vi "GROUND cube sat.vi"() -> ()   [LabVIEW 2020]
uses:
  <vilib>/Utility/file.llb/Write Delimited Spreadsheet (string).vi
  <vilib>/Instr/_visa.llb/VISA Configure Serial Port (Instr).vi
panel:
  out "after BMP":string
  in  "read buffer":string
  in  "Tab Control":enum32{"Page 1", "Page 2"}(tab)
  out "Sensor ID":string
  out "SSTL":string
  out "AER":string
  in  "?":bool
  out "result":bool
  in  "?":T1(tab)
  out "RIGHT DATA":bool
  out "WRONG DATA":bool
  out "True password":bool
  in  "file path (dialog if empty) 2":path
  in  "VISA resource name":refnum<visa-resource-name>
  in  "Password":string
  in  "Username":string
  in  "OK":bool
  out "msg":string
  out "String":string
  in  "Send command":bool
  in  "velocity":dbl
  in  "distance":dbl
  out "time":dbl
  out "BMP Temprature (C)":dbl(slide) scale=0.0..100.0
  out "Altitude (m)":dbl(slide) scale=0.0..100000.0
  out "Pressure (Pa)":dbl(knob) scale=0.0..101325.0
  out "Altitude(m)":dbl
  out "Pressure(Pa)":dbl
  out "Temperature(C)":dbl
  out "Reads_BMP":string
  out "BMP_CRC WORKING":bool
  out "DHT temp (C)":dbl(slide) scale=-100.0..100.0
  out "DHT humidity (%)":dbl(knob) scale=0.0..100.0
  out "DHT temp(C)":dbl
  out "DHT humidity(%)":dbl
  out "Reads_DHT":string
  out "DHT_CRC WORKING":bool
  out "accel_z":dbl(slide) scale=0.0..1000.0
  out "accel_y":dbl(slide) scale=0.0..1000.0
  out "accel_x":dbl(slide) scale=0.0..1000.0
  out "phi":dbl(slide) scale=0.0..360.0
  out "theta":dbl(slide) scale=0.0..360.0
  out "psi":dbl(slide) scale=0.0..360.0
  out "FILTERD SIGNALS":dynamicdata(graph)
  out "SIGNALS":dynamicdata(graph)
  out "accel_x (m/s^2)":dbl
  out "accel_z(m/s^2)":dbl
  out "accel_y(m/s^2)":dbl
  out "phi":dbl
  out "psi":dbl
  out "theta":dbl
  in  "?":bool
  in  "Start Filtering":bool
  out "Reads_MPU":string
  out "MPU_CRC WORKING":bool
  out "ALT":i32
  in  "Zoom":sgl=16.0 format="%#.1g"
  in  "Size Y":dbl=650.0
  in  "Size X":dbl=450.0
  in  "Map Format":string(combo)="roadmap"
  out "LAT":i32
  out "LONG":i32
  in  "WebBrowser":refnum<k7>(container)
  out "ID":string
  out "Reads_GPS":string
  out "GPS_CRC WORKING":bool
  out "Image Out":T2(plugin-control)
  in  "Contrast::Value":dbl=0.32 min=0.0 max=0.64
  in  "Bayer::Gain R":dbl=1.0 min=0.0 max=3.999
  in  "Hue::Value":dbl min=-0.4 max=0.4
  in  "Bayer::Gain B":dbl=1.0 min=0.0 max=3.999
  in  "Bayer::Gain G":dbl=1.0 min=0.0 max=3.999
  out "pic number":dbl
  in  "Stop (F)":bool
  out "Time":string
  in  "Gamma::Value":dbl=1.0 min=0.72 max=5.0
  in  "Brightness::Value":i64 min=-64 max=64 step=1
  in  "Sharpness::Value":i64 min=0 max=5 step=1
  in  "Saturation::Value":i64=64 min=0 max=128 step=1
  in  "Take pic":bool
  in  "path":string
  # "The Cube sat"
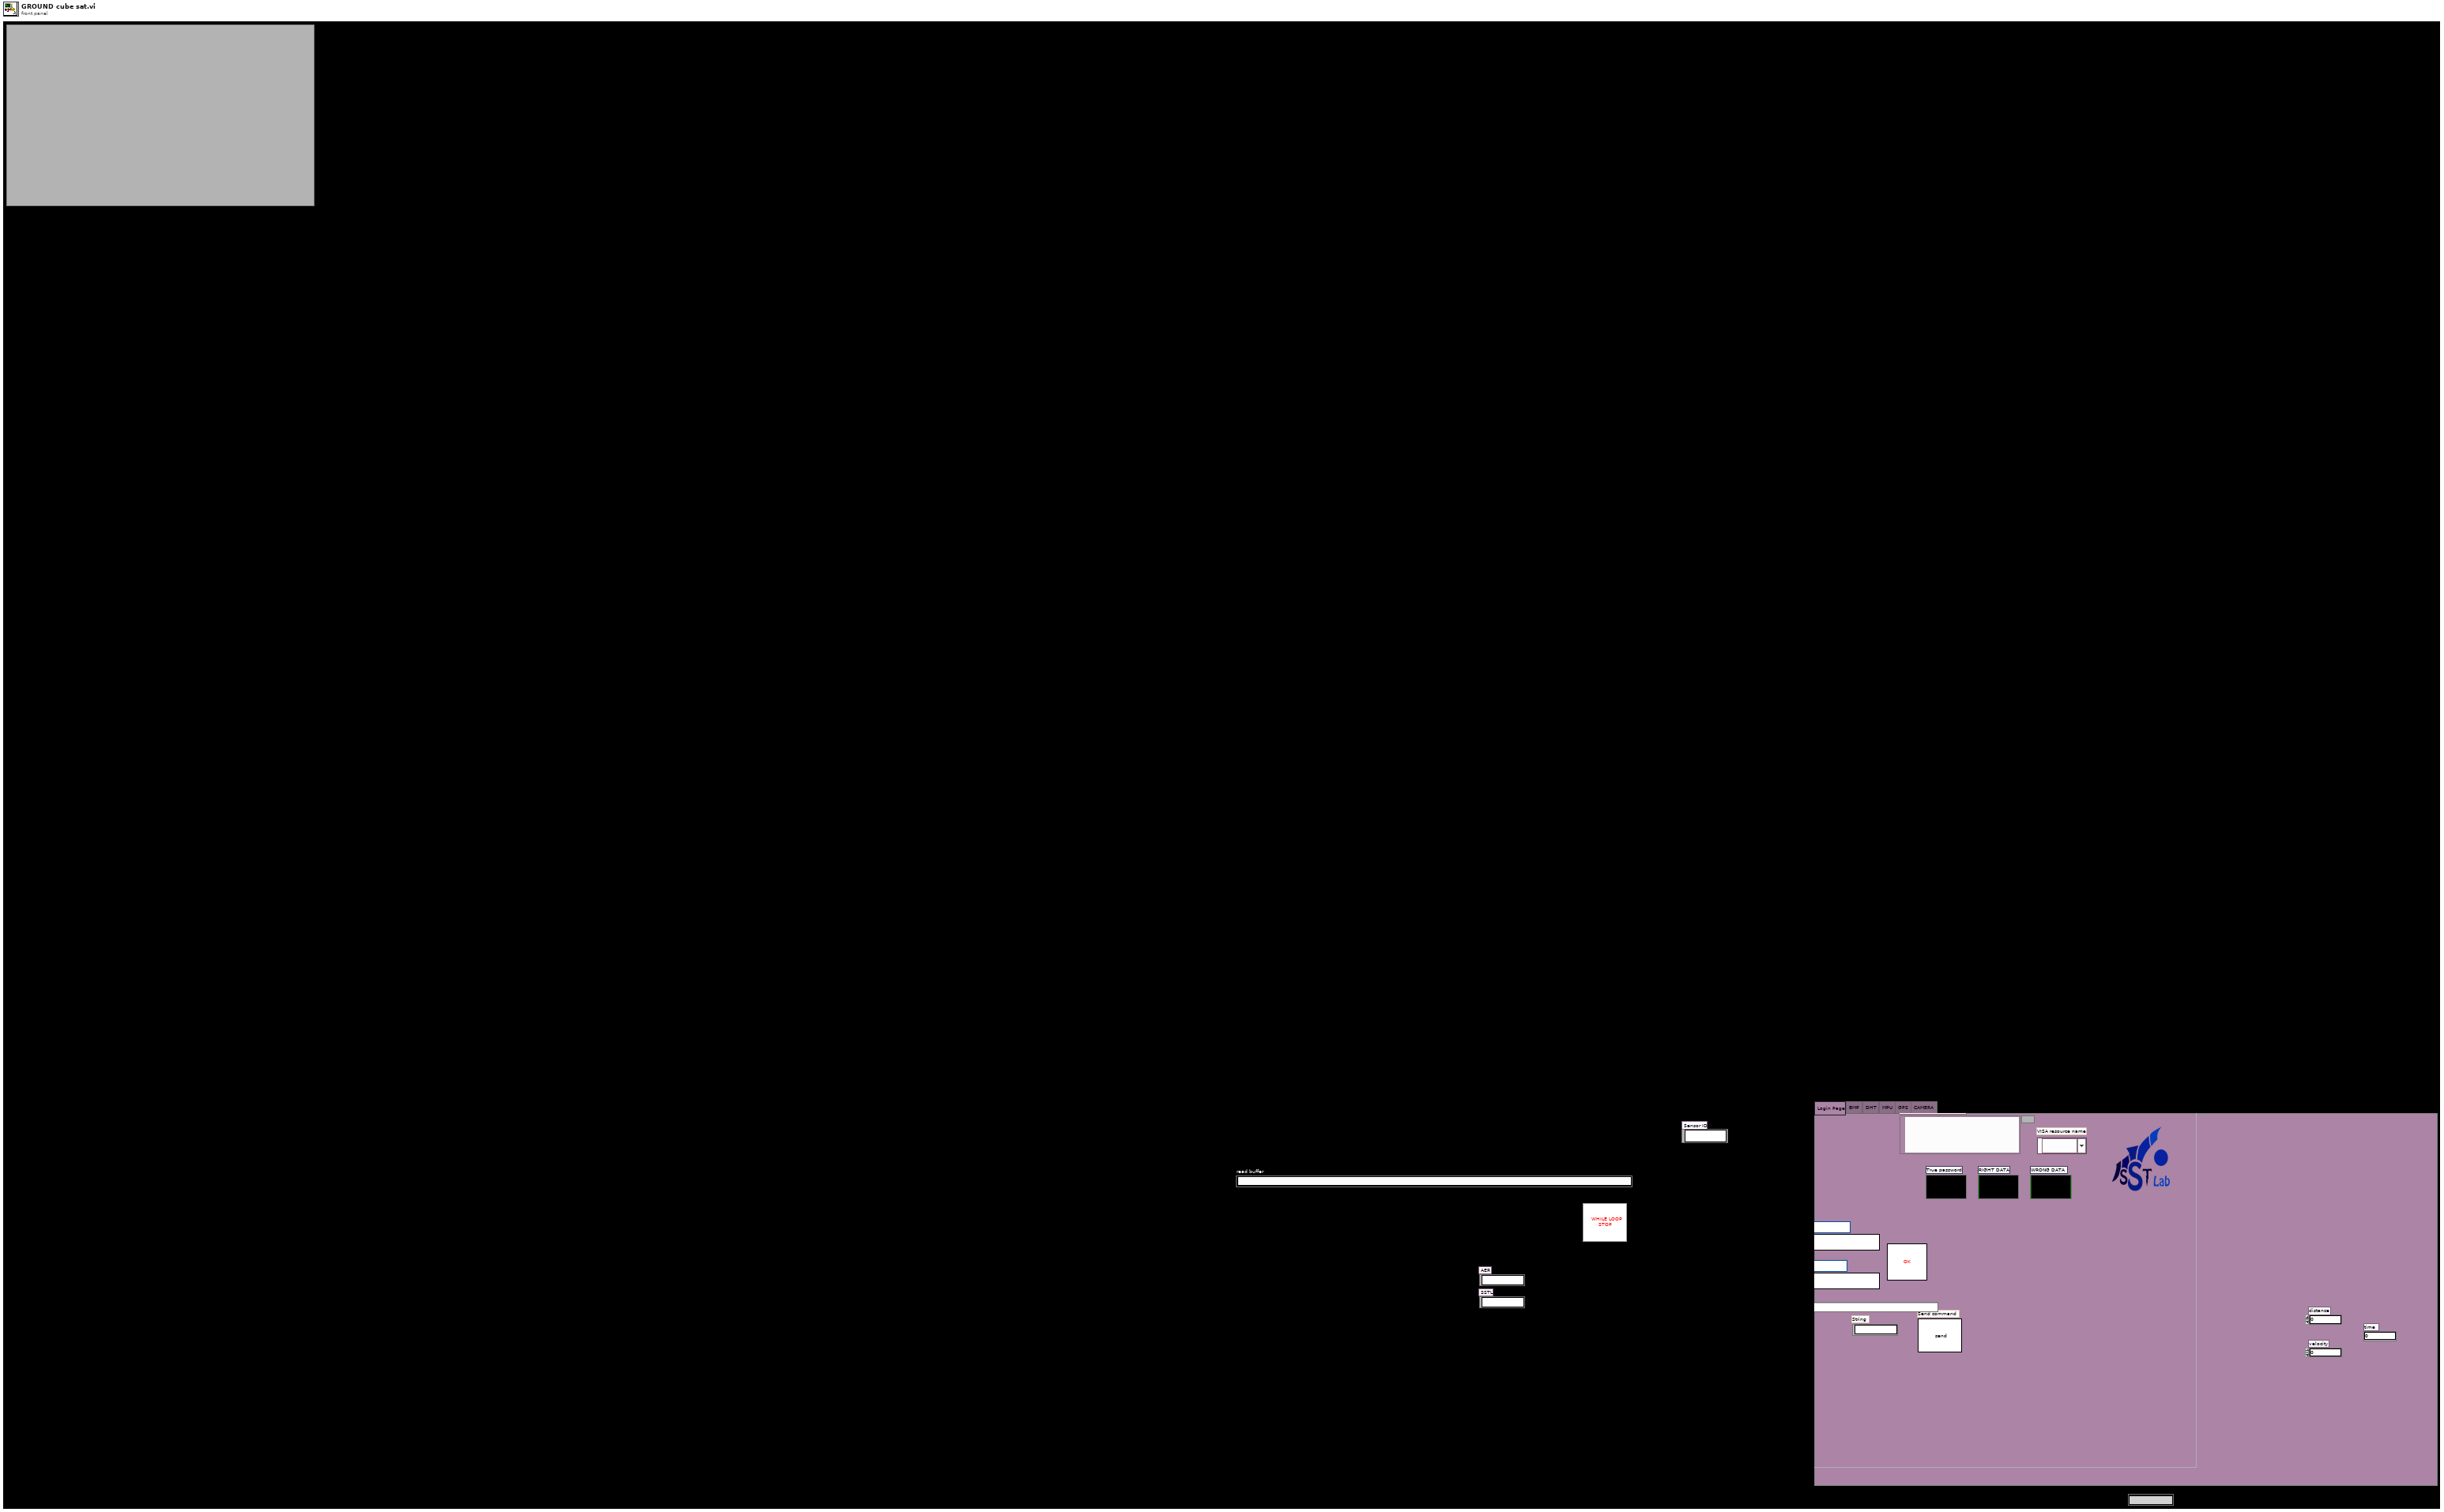
[diagram p1: front panel]
types:
  T1 = enum32{"Login Page", "BMP", "DHT", "MPU", "GPS", "CAMERA"}
  T2 = typedef "IMAQ Image.ctl" = refnum<image>
  T3 = enum32{"Page 1", "Page 2", "Page 3", "Page 4", "Page 5", "Page 6"}
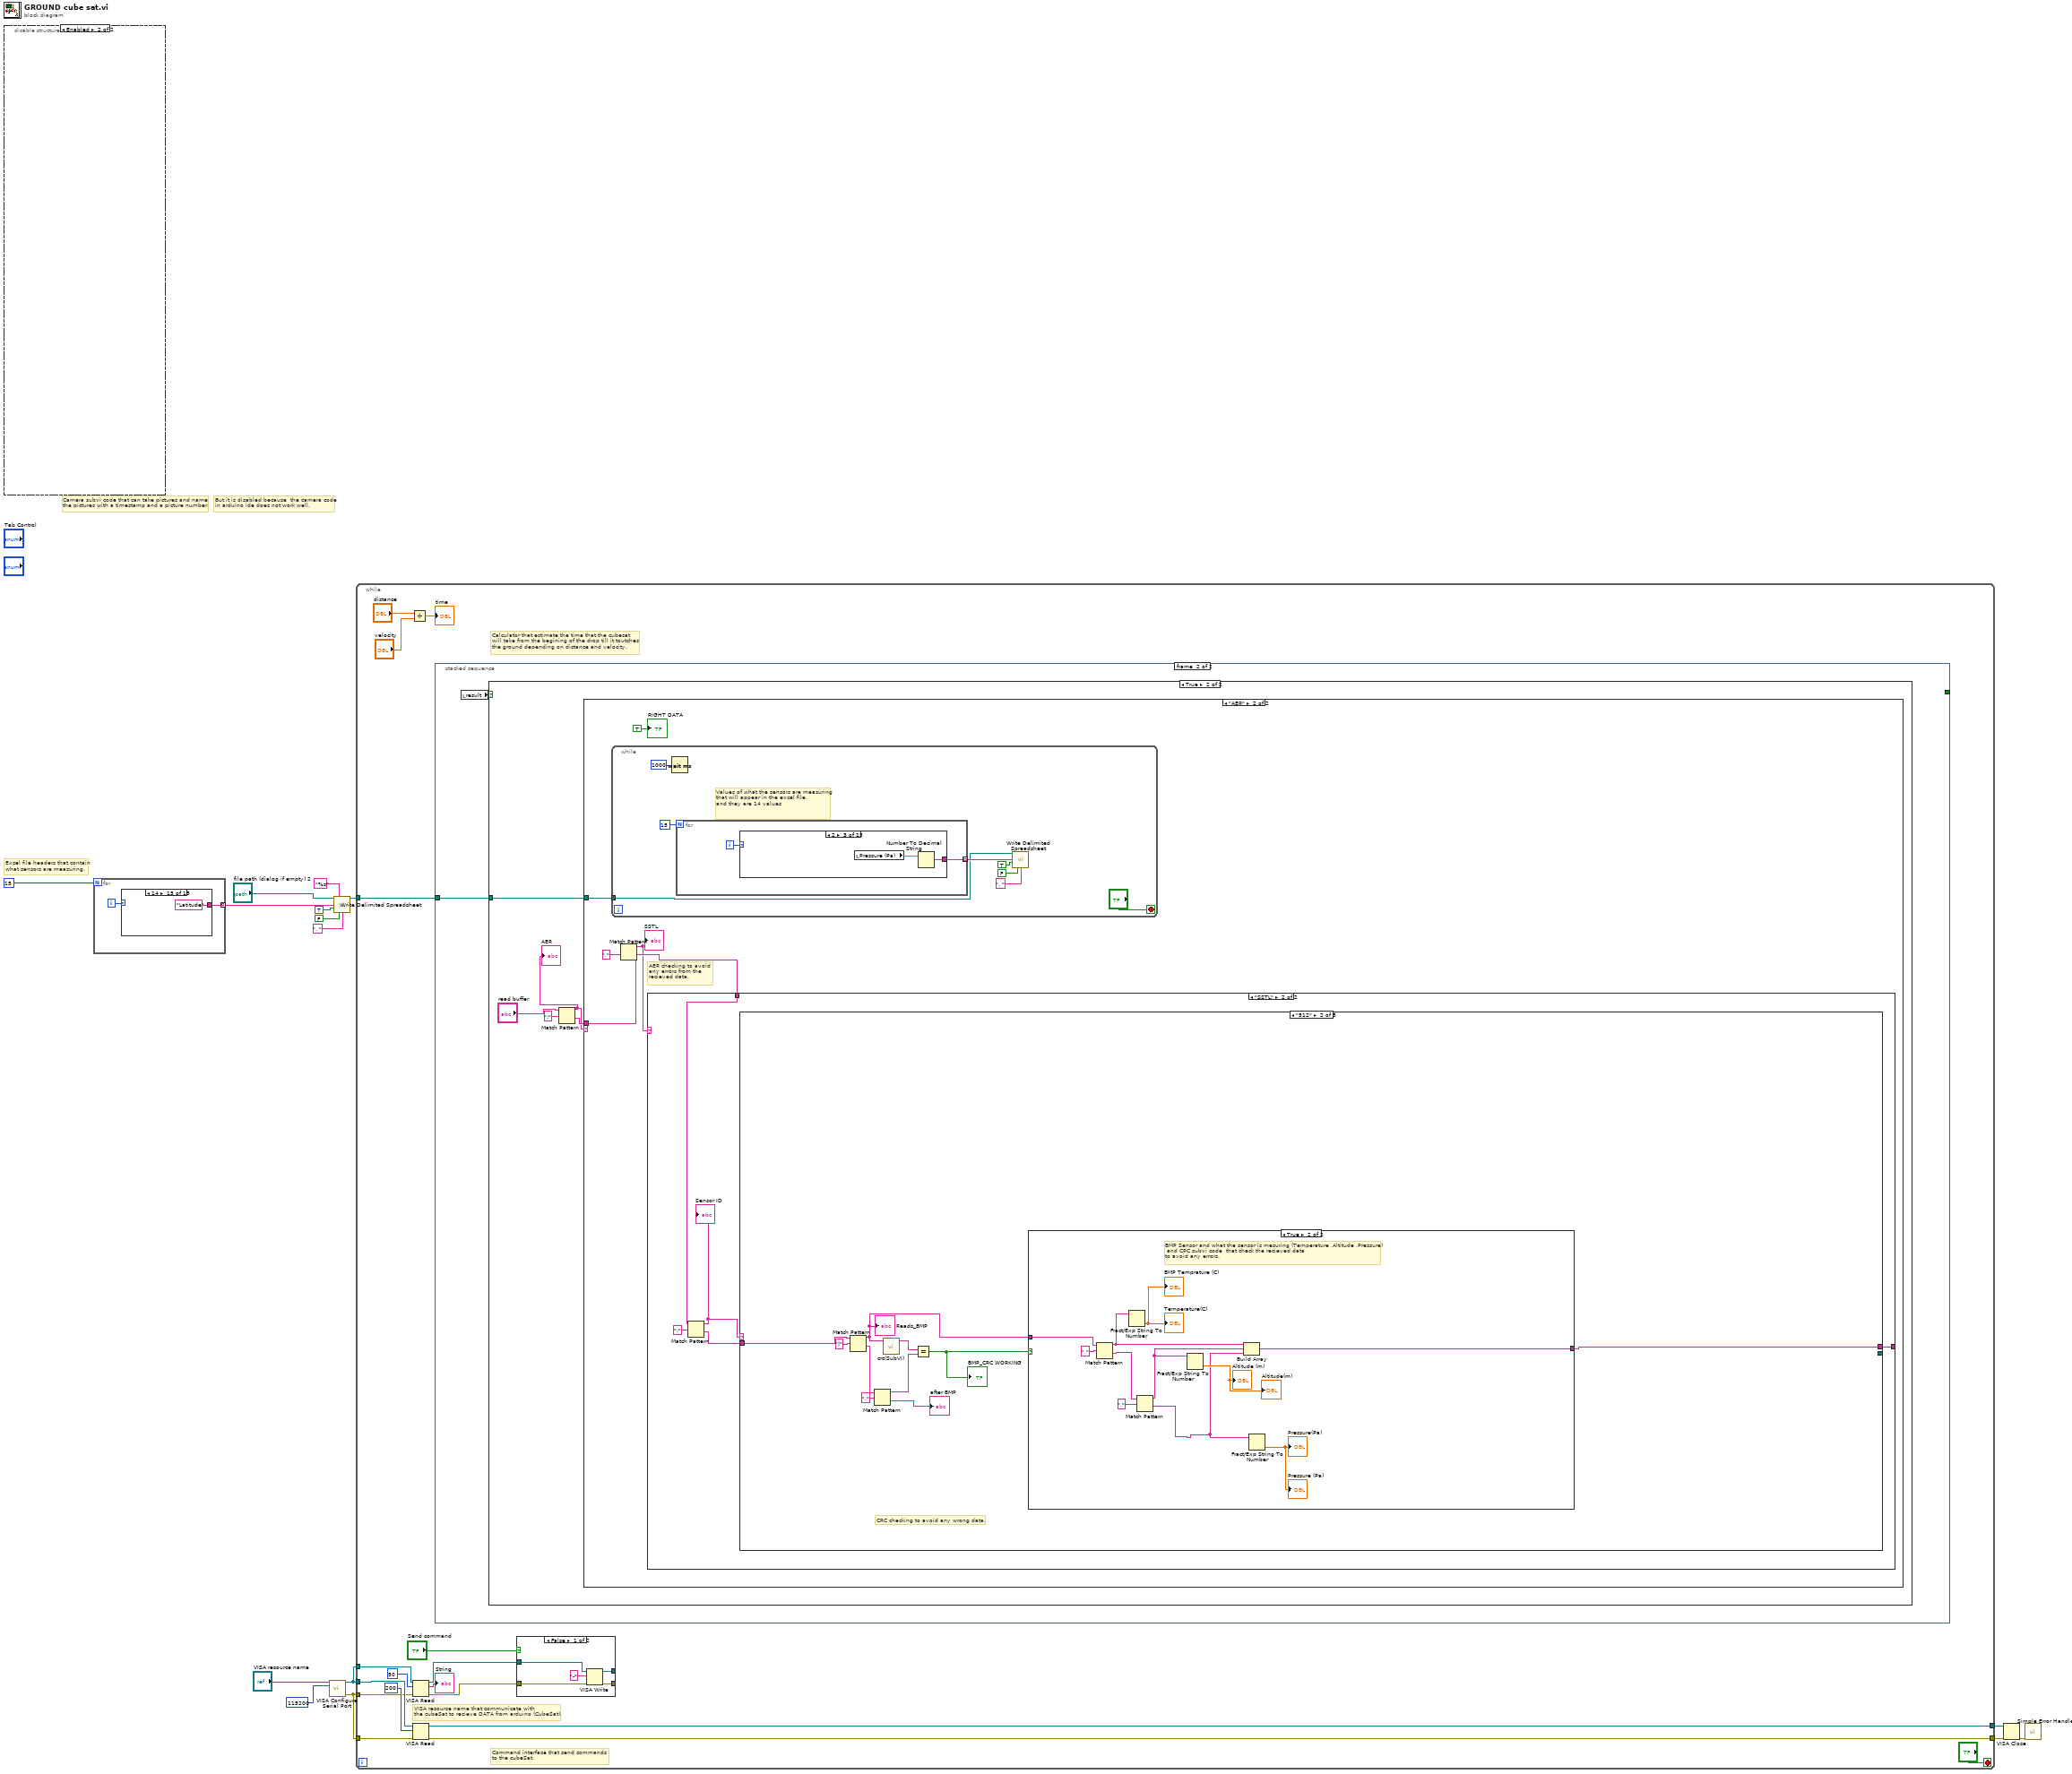
[diagram p0: block diagram]
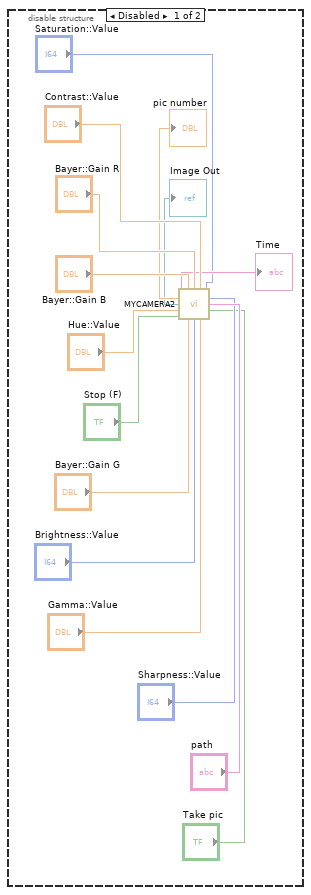
[diagram p2: hidden frame]
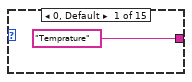
[diagram p3: hidden frame]
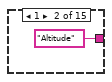
[diagram p4: hidden frame]
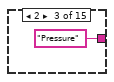
[diagram p5: hidden frame]
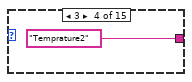
[diagram p6: hidden frame]
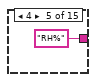
[diagram p7: hidden frame]
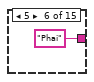
[diagram p8: hidden frame]
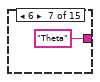
[diagram p9: hidden frame]
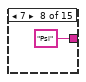
[diagram p10: hidden frame]
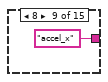
[diagram p11: hidden frame]
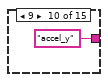
[diagram p12: hidden frame]
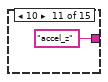
[diagram p13: hidden frame]
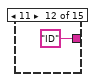
[diagram p14: hidden frame]
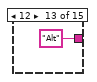
[diagram p15: hidden frame]
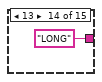
[diagram p16: hidden frame]
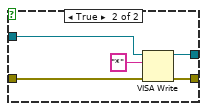
[diagram p17: hidden frame]
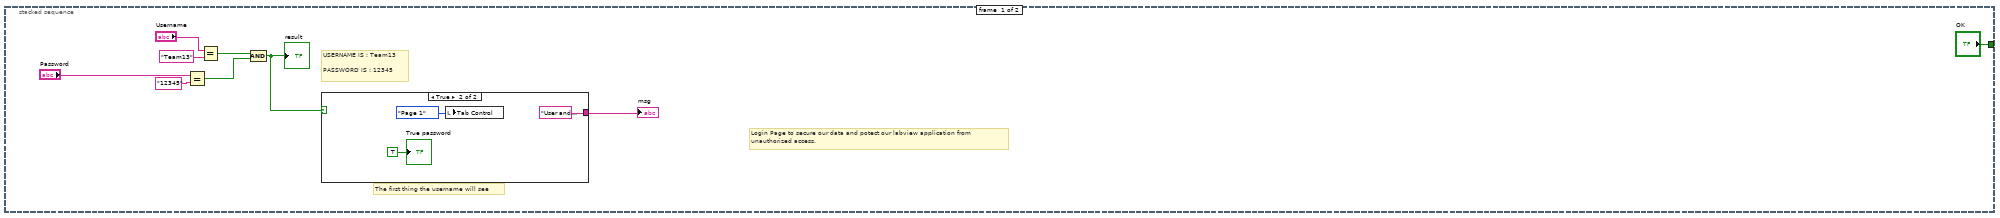
[diagram p18: hidden frame]
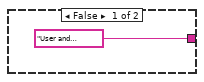
[diagram p19: hidden frame]
diagram:
  # "But it is disabled because  the camera code \nin arduino ide does not work well."
  # "Excel file headers that contain\nwhat sensors are measuring."
  # "Camera subvi code that can take pictures and name \nthe pictures with a timestamp and a picture number."
  n1 = disable-structure shown="Enabled" {
    frame Disabled {
      n2 = call "MYCAMERA2.vi"("Bayer::Gain B"="Bayer::Gain B", "Bayer::Gain R"="Bayer::Gain R", "Contrast::Value"="Contrast::Value", "Saturation::Value"="Saturation::Value", "Sharpness::Value"="Sharpness::Value", "path"="path", "Hue::Value"="Hue::Value", "Take pic"="Take pic", "Stop (F)"="Stop (F)", "Bayer::Gain G"="Bayer::Gain G", "Brightness::Value"="Brightness::Value", "Gamma::Value"="Gamma::Value") -> ("Time"=→"Time":string, "pic number"=→"pic number":dbl, "Image Out"=→"Image Out":T2)  [unwired: 1 in]
    }
    frame Enabled {
    }
  }
  n3 = for {
    N: 15 -> [_]
    tunnel: [w31] -> w15 mode=indexing
    i -> [w32]
    n4 = case shown="14" w32 {
      tunnel: ["Temprature" "Altitude" "Pressure" "Temprature2" "RH%" "Phai" "Theta" "Psi" "accel_x" "accel_y" "accel_z" "ID" "Alt" "LONG" "Latitude"] -> w31
      frame 0, Default {
      }
      frame 1 {
      }
      frame 2 {
      }
      frame 3 {
      }
      frame 4 {
      }
      frame 5 {
      }
      frame 6 {
      }
      frame 7 {
      }
      frame 8 {
      }
      frame 9 {
      }
      frame 10 {
      }
      frame 11 {
      }
      frame 12 {
      }
      frame 13 {
      }
      frame 14 {
      }
    }
  }
  n5 = call-poly "VISA Configure Serial Port"("VISA resource name"="VISA resource name", "baud rate (9600)"=u32 115200) -> ("VISA resource name out"=w2:refnum<visa-resource-name>, "error out"=w1:errorcluster)  [unwired: 12 in]
  n6 = call-poly <vilib>:"Write Delimited Spreadsheet.vi"("file path (dialog if empty)"="file path (dialog if empty) 2", "format (%s)"="%s", "1D data"=w15, "append to file? (new file:F)"=TRUE, "transpose? (no:F)"=FALSE, "delimiter (\\t)"=", " ("delimiter (\\t)")) -> ("new file path (Not A Path if cancelled)"=w8:path)  [unwired: 8 in, 1 out]
  n7 = while {
    tunnel: w8 -> [w55]
    tunnel: w2 -> [w53]
    tunnel: w1 -> [w52]
    tunnel: [w51] -> w4
    tunnel: [w50] -> w3
    tunnel: w2 -> [w49]
    tunnel: w1 -> [w48]
    stop <- "?" stop-if-true
    # "Command interface that send commands \nto the cubeSat."
    # "Calculator that estimate the time that the cubesat \nwill take from the begining of the drop till it toutches \nthe ground depending on distance and velocity."
    # "VISA resourse name that communicate with \nthe cubeSat to recieve DATA from arduino (CubeSat)."
    n8 = Divide(x="distance", y="velocity") -> (x/y=→"time":dbl)
    n9 = VISA Read(VISA resource name=w49, byte count=u32 50, error in (no error)=w48) -> (VISA resource name out=w61:refnum<visa-resource-name>, read buffer=→"String":string, error out=w62:errorcluster)  [unwired: 1 out]
    n10 = VISA Read(VISA resource name=w53, byte count=u32 200, error in (no error)=w52) -> (VISA resource name out=w50:refnum<visa-resource-name>, error out=w51:errorcluster)  [unwired: 2 out]
    n11 = stacked-sequence {
      tunnel: ["OK" _] -> _
      tunnel: w55 -> [_ w88]
      frame #0 {
        # "USERNAME IS : Team13\n\nPASSWORD IS : 12345"
        # "The first thing the username will see"
        # "Login Page to secure our data and potect our labview application from \nunauthorized access."
        n12 = Equal?(x="Password", y="12345") -> (x = y?=w76:bool)
        n13 = Equal?(x="Username", y="Team13") -> (x = y?=w80:bool)
        n14 = Compound Arithmetic op=AND(w80, w76) -> (w83:bool)
        "result" <- w83
        n15 = case shown="True" w83 {
          tunnel: ["User and password are False" "User and Password ara True"] -> w82
          frame False {
          }
          frame True {
            n16 = local write "Tab Control"(T3."Page 1" ("Tab Control")) -> ()
            "True password" <- TRUE ("Boolean 2")
          }
        }
        "msg" <- w82
      }
      frame #1 {
        n17 = local read "result"() -> (w89:bool)
        n18 = case shown="True" w89 {
          tunnel: w88 -> [_ w94]
          frame False {
          }
          frame True {
            n19 = Match Pattern(string="read buffer", regular expression=":") -> (before substring=w90:string, after substring=w91:string)  [unwired: 1 in, 2 out]
            "AER" <- w90
            n20 = case shown="\"AER\"" w90 {
              tunnel: w94 -> [_ w101]
              tunnel: w91 -> [_ w99]
              frame "False", Default {
                "WRONG DATA" <- TRUE ("Boolean")
              }
              frame "AER" {
                # "AER checking to avoid \nany errors from the \nrecieved data."
                n21 = while {
                  tunnel: w101 -> [w105]
                  stop <- "?" stop-if-true
                  # "Values of what the sensors are measuring\nthat will appear in the excel file. \nand they are 14 values"
                  n22 = Wait (ms)(milliseconds to wait=u32 1000) -> ()  [unwired: 1 out]
                  n23 = for {
                    N: 15 -> [_]
                    tunnel: [w110] -> w106 mode=indexing
                    i -> [w111]
                    n24 = case shown="2" w111 {
                      tunnel: [w112 w114 w116 w118 w120 w122 w124 w126 w128 w130 w132 w134 w136 w137 w139] -> w110
                      frame 0, Default {
                        n25 = local read "BMP Temprature (C)"() -> (w113:dbl)
                        n26 = Number To Decimal String(number=w113) -> (decimal integer string=w112:string)  [unwired: 1 in]
                      }
                      frame 1 {
                        n27 = local read "Altitude (m)"() -> (w115:dbl)
                        n28 = Number To Decimal String(number=w115) -> (decimal integer string=w114:string)  [unwired: 1 in]
                      }
                      frame 2 {
                        n29 = local read "Pressure (Pa)"() -> (w117:dbl)
                        n30 = Number To Decimal String(number=w117) -> (decimal integer string=w116:string)  [unwired: 1 in]
                      }
                      frame 3 {
                        n31 = local read "DHT temp (C)"() -> (w119:dbl)
                        n32 = Number To Decimal String(number=w119) -> (decimal integer string=w118:string)  [unwired: 1 in]
                      }
                      frame 4 {
                        n33 = local read "DHT humidity (%)"() -> (w121:dbl)
                        n34 = Number To Decimal String(number=w121) -> (decimal integer string=w120:string)  [unwired: 1 in]
                      }
                      frame 5 {
                        n35 = local read "phi"() -> (w123:dbl)
                        n36 = Number To Decimal String(number=w123) -> (decimal integer string=w122:string)  [unwired: 1 in]
                      }
                      frame 6 {
                        n37 = local read "theta"() -> (w125:dbl)
                        n38 = Number To Decimal String(number=w125) -> (decimal integer string=w124:string)  [unwired: 1 in]
                      }
                      frame 7 {
                        n39 = local read "psi"() -> (w127:dbl)
                        n40 = Number To Decimal String(number=w127) -> (decimal integer string=w126:string)  [unwired: 1 in]
                      }
                      frame 8 {
                        n41 = local read "accel_x"() -> (w129:dbl)
                        n42 = Number To Decimal String(number=w129) -> (decimal integer string=w128:string)  [unwired: 1 in]
                      }
                      frame 9 {
                        n43 = local read "accel_y"() -> (w131:dbl)
                        n44 = Number To Decimal String(number=w131) -> (decimal integer string=w130:string)  [unwired: 1 in]
                      }
                      frame 10 {
                        n45 = local read "accel_z"() -> (w133:dbl)
                        n46 = Number To Decimal String(number=w133) -> (decimal integer string=w132:string)  [unwired: 1 in]
                      }
                      frame 11 {
                        n47 = local read "ID"() -> (w134:string)
                      }
                      frame 12 {
                        n48 = local read "ALT"() -> (w135:i32)
                        n49 = Number To Decimal String(number=w135) -> (decimal integer string=w136:string)  [unwired: 1 in]
                      }
                      frame 13 {
                        n50 = local read "LONG"() -> (w138:i32)
                        n51 = Number To Decimal String(number=w138) -> (decimal integer string=w137:string)  [unwired: 1 in]
                      }
                      frame 14 {
                        n52 = local read "LAT"() -> (w140:i32)
                        n53 = Number To Decimal String(number=w140) -> (decimal integer string=w139:string)  [unwired: 1 in]
                      }
                    }
                  }
                  n54 = call-poly <vilib>:"Write Delimited Spreadsheet.vi"("file path (dialog if empty)"=w105, "1D data"=w106, "append to file? (new file:F)"=TRUE, "transpose? (no:F)"=FALSE, "delimiter (\\t)"=", " ("delimiter (\\t)")) -> ()  [unwired: 9 in, 2 out]
                }
                n55 = Match Pattern(string=w99, regular expression=",") -> (before substring=w96:string, after substring=w97:string)  [unwired: 1 in, 2 out]
                "SSTL" <- w96
                n56 = case shown="\"SSTL\"" w96 {
                  tunnel: [_ w145] -> _
                  tunnel: w97 -> [_ w144]
                  frame "False", Default {
                  }
                  frame "SSTL" {
                    n57 = Match Pattern(string=w144, regular expression=":") -> (before substring=w141:string, after substring=w142:string)  [unwired: 1 in, 2 out]
                    "Sensor ID" <- w141
                    n58 = case shown="\"512\"" w141 {
                      tunnel: [_ w156 w176 w192 _] -> w145
                      tunnel: [_ _ _ _ w234] -> _
                      tunnel: w142 -> [_ w152 w173 w188 w230]
                      frame "0", Default {
                        n59 = local write "WRONG DATA"(TRUE ("Boolean")) -> ()
                      }
                      frame "512" {
                        # "CRC checking to avoid any wrong data."
                        n60 = Match Pattern(string=w152, regular expression="|") -> (before substring=w155:string, after substring=w151:string)  [unwired: 1 in, 2 out]
                        "Reads_BMP" <- w155
                        n61 = Match Pattern(string=w151, regular expression=",") -> (before substring=w149:string, after substring=→"after BMP":string)  [unwired: 1 in, 2 out]
                        n62 = call "crc(SubVI).vi"("String"=w155) -> ("CRC-16 MODBUS Byte Swap 2"=w153:string)  [unwired: 10 in]
                        n63 = Equal?(x=w153, y=w149) -> (x = y?=w147:bool)
                        "BMP_CRC WORKING" <- w147
                        n64 = case shown="True" w147 {
                          tunnel: [_ w159] -> w156
                          tunnel: w155 -> [_ w158]
                          frame False {
                          }
                          frame True {
                            # "BMP Sensor and what the sensor is mesuring (Temperature ,Altitude ,Pressure)\n and CRC subvi code  that check the recieved data\nto avoid any errors."
                            n65 = Match Pattern(string=w158, regular expression=",") -> (before substring=w161:string, after substring=w165:string)  [unwired: 1 in, 2 out]
                            n66 = Fract/Exp String To Number(string=w161) -> (number=→"BMP Temprature (C)" →"Temperature(C)":dbl)  [unwired: 3 in, 1 out]
                            n67 = Match Pattern(string=w165, regular expression=",") -> (before substring=w160:string, after substring=w157:string)  [unwired: 1 in, 2 out]
                            n68 = Fract/Exp String To Number(string=w160) -> (number=→"Altitude (m)" →"Altitude(m)":dbl)  [unwired: 3 in, 1 out]
                            n69 = Build Array(w161, w160, w157) -> (w159:string[])
                            n70 = Fract/Exp String To Number(string=w157) -> (number=→"Pressure (Pa)" →"Pressure(Pa)":dbl)  [unwired: 3 in, 1 out]
                          }
                        }
                      }
                      frame "513" {
                        # "CRC checking to avoid any wrong data."
                        n71 = Match Pattern(string=w173, regular expression="|") -> (before substring=w172:string, after substring=w171:string)  [unwired: 1 in, 2 out]
                        "Reads_DHT" <- w172
                        n72 = Match Pattern(string=w171, regular expression=",") -> (before substring=w169:string)  [unwired: 1 in, 3 out]
                        n73 = call "crc(SubVI).vi"("String"=w172) -> ("CRC-16 MODBUS Byte Swap 2"=w174:string)  [unwired: 10 in]
                        n74 = Equal?(x=w174, y=w169) -> (x = y?=w168:bool)
                        "DHT_CRC WORKING" <- w168
                        n75 = case shown="True" w168 {
                          tunnel: [_ w179] -> w176
                          tunnel: w172 -> [_ w178]
                          frame False {
                          }
                          frame True {
                            # "DHT sensor and what the sensor is measuring (Temperature and humidity) \nand CRC subvi code  that check the recieved data\nto avoid any errors."
                            n76 = Match Pattern(string=w178, regular expression=",") -> (before substring=w180:string, after substring=w177:string)  [unwired: 1 in, 2 out]
                            n77 = Fract/Exp String To Number(string=w180) -> (number=→"DHT temp (C)" →"DHT temp(C)":dbl)  [unwired: 3 in, 1 out]
                            n78 = Build Array(w180, w177) -> (w179:string[])
                            n79 = Fract/Exp String To Number(string=w177) -> (number=→"DHT humidity (%)" →"DHT humidity(%)":dbl)  [unwired: 3 in, 1 out]
                          }
                        }
                      }
                      frame "514" {
                        # "CRC checking to avoid any wrong data."
                        n80 = Match Pattern(string=w188, regular expression="|") -> (before substring=w191:string, after substring=w187:string)  [unwired: 1 in, 2 out]
                        "Reads_MPU" <- w191
                        n81 = call "crc(SubVI).vi"("String"=w191) -> ("CRC-16 MODBUS Byte Swap 2"=w189:string)  [unwired: 10 in]
                        n82 = Match Pattern(string=w187, regular expression=",") -> (before substring=w185:string)  [unwired: 1 in, 3 out]
                        n83 = Equal?(x=w189, y=w185) -> (x = y?=w184:bool)
                        "MPU_CRC WORKING" <- w184
                        n84 = case shown="True" w184 {
                          tunnel: [_ w209] -> w192
                          tunnel: w191 -> [_ w197]
                          frame False {
                          }
                          frame True {
                            # "An option  to apply a filter on the received MPU data \nto reduce noise and smooth the signal."
                            # "MPU sensor and what the sensor is measuring:\" ANGLES\" (phi , theta , psi) and \n \" Acceleration over the X ,Y and Z axis\".\n CRC subvi code  that check the recieved data\nto avoid any errors."
                            n85 = Match Pattern(string=w197, regular expression=",") -> (before substring=w214:string, after substring=w219:string)  [unwired: 1 in, 2 out]
                            n86 = Fract/Exp String To Number(string=w214) -> (number=w200:dbl)  [unwired: 3 in, 1 out]
                            "phi" <- w200
                            "phi" <- w200
                            n87 = Match Pattern(string=w219, regular expression=",") -> (before substring=w213:string, after substring=w223:string)  [unwired: 1 in, 2 out]
                            n88 = Fract/Exp String To Number(string=w213) -> (number=w199:dbl)  [unwired: 3 in, 1 out]
                            "theta" <- w199
                            "theta" <- w199
                            n89 = Match Pattern(string=w223, regular expression=",") -> (before substring=w212:string, after substring=w218:string)  [unwired: 1 in, 2 out]
                            n90 = call "Simulate Signal"("Frequency"=10.0, "Amplitude"=w200) -> ("Sine"=w208:dynamicdata)  [unwired: 12 in, 1 out]
                            n91 = Fract/Exp String To Number(string=w212) -> (number=w198:dbl)  [unwired: 3 in, 1 out]
                            "psi" <- w198
                            "psi" <- w198
                            n92 = Match Pattern(string=w218, regular expression=",") -> (before substring=w210:string, after substring=w217:string)  [unwired: 1 in, 2 out]
                            n93 = call "Simulate Signal2"("Frequency"=10.0, "Amplitude"=w199) -> ("Sine"=w205:dynamicdata)  [unwired: 12 in, 1 out]
                            n94 = Fract/Exp String To Number(string=w210) -> (number=→"accel_x" →"accel_x (m/s^2)":dbl)  [unwired: 3 in, 1 out]
                            n95 = Match Pattern(string=w217, regular expression=",") -> (before substring=w211:string, after substring=w193:string)  [unwired: 1 in, 2 out]
                            n96 = call "Simulate Signal3"("Frequency"=10.0, "Amplitude"=w198) -> ("Sine"=w204:dynamicdata)  [unwired: 12 in, 1 out]
                            n97 = Fract/Exp String To Number(string=w211) -> (number=→"accel_y" →"accel_y(m/s^2)":dbl)  [unwired: 3 in, 1 out]
                            n98 = Fract/Exp String To Number(string=w193) -> (number=→"accel_z" →"accel_z(m/s^2)":dbl)  [unwired: 3 in, 1 out]
                            n99 = Build Array(w214, w213, w212, w210, w211, w193) -> (w209:string[])
                            n100 = Merge Signals(w208, w205, w204) -> (w203:dynamicdata)
                            "SIGNALS" <- w203
                            n101 = case shown="True" "Start Filtering" {
                              tunnel: w203 -> [_ w225]
                              frame False {
                              }
                              frame True {
                                n102 = call "Filter"("Signal"=w225) -> ("Filtered Signal"=→"FILTERD SIGNALS":dynamicdata)  [unwired: 9 in, 1 out]
                              }
                            }
                          }
                        }
                      }
                      frame "515" {
                        # "CRC checking to avoid any wrong data."
                        n103 = Match Pattern(string=w230, regular expression="|") -> (before substring=w233:string, after substring=w229:string)  [unwired: 1 in, 2 out]
                        "Reads_GPS" <- w233
                        n104 = Match Pattern(string=w229, regular expression=",") -> (before substring=w227:string)  [unwired: 1 in, 3 out]
                        n105 = call "crc(SubVI).vi"("String"=w233) -> ("CRC-16 MODBUS Byte Swap 2"=w231:string)  [unwired: 10 in]
                        n106 = Equal?(x=w231, y=w227) -> (x = y?=w226:bool)
                        "GPS_CRC WORKING" <- w226
                        n107 = case shown="True" w226 {
                          tunnel: [_ w253] -> w234
                          tunnel: w233 -> [_ w251]
                          frame False {
                          }
                          frame True {
                            w246 = " AIzaSyBu-916DdpKAjTmJNIgngS6HL_kDIKU0aU"  # Google Maps API Key
                            # "GPS sensor and what the sensor is measuring ( Lattitude , longitude , ID ,Altitude )) \nand CRC subvi code  that check the recieved data\nto avoid any errors."
                            n108 = Match Pattern(string=w251, regular expression=",") -> (before substring=→"ID":string, after substring=w252:string)  [unwired: 1 in, 2 out]
                            n109 = Match Pattern(string=w252, regular expression=",") -> (before substring=w250:string, after substring=w257:string)  [unwired: 1 in, 2 out]
                            n110 = Match Pattern(string=w257, regular expression=",") -> (before substring=w249:string, after substring=w236:string)  [unwired: 1 in, 2 out]
                            n111 = Decimal String To Number(string=w250) -> (number=→"ALT":i32)  [unwired: 2 in, 1 out]
                            n112 = Decimal String To Number(string=w236) -> (number=w235:i32)  [unwired: 2 in, 1 out]
                            "LAT" <- w235
                            n113 = Decimal String To Number(string=w249) -> (offset past number=w237:i32)  [unwired: 2 in, 1 out]
                            "LONG" <- w237
                            n114 = call "Create Map URL.vi"("Map Format"="Map Format", "X"="Size X", "Lat"=w235, "Y"="Size Y", "Zoom"="Zoom", "Lon"=w237) -> ("String"=w240:string)  [unwired: 5 in]
                            n115 = Concatenate Strings(w240, "&markers=" ("string"), "color:" ("string"), "Red" ("color"), "%7C" ("string"), "label:" ("string"), "Team13" ("string"), "%7C" ("string"), "," ("string"), "&key=" ("string"), w246) -> (w258:string)
                            n116 = invoke class="IWebBrowser2" method="Navigate"(reference="WebBrowser", "URL"=w258) -> (reference out=w253:refnum<k7>)  [unwired: 6 in, 7 out]
                          }
                        }
                      }
                    }
                  }
                }
                "RIGHT DATA" <- TRUE ("GREEN")
              }
            }
          }
        }
      }
    }
    n117 = case shown="False" "Send command" {
      tunnel: w61 -> [w67 w74]
      tunnel: [w66 w73] -> _
      tunnel: w62 -> [w68 w72]
      tunnel: [w65 w71] -> _
      frame False {
        n118 = VISA Write(VISA resource name=w67, write buffer="-", error in (no error)=w68) -> (VISA resource name out=w66:refnum<visa-resource-name>, error out=w65:errorcluster)  [unwired: 1 out]
      }
      frame True {
        n119 = VISA Write(VISA resource name=w74, write buffer="*", error in (no error)=w72) -> (VISA resource name out=w73:refnum<visa-resource-name>, error out=w71:errorcluster)  [unwired: 1 out]
      }
    }
  }
  n120 = VISA Close(VISA resource name=w3, error in (no error)=w4) -> (error out=w5:errorcluster)
  n121 = call <vilib>:"Simple Error Handler.vi"("error in (no error)"=w5) -> ()  [unwired: 4 in, 5 out]
